vi "Automated door project by Rinat.vi"() -> ()   [LabVIEW 2020]
panel:
  out "String 2":string
  out "String":string
  in  "stop":bool
  out "Door 2":dbl(slide)
  in  "Distance from the door":dbl(knob) scale=0.2..3.0
  out "Door":dbl(slide) scale=0.0..100.0
  out "Door Motor (Closing)":bool
  out "Door Motor (Opening)":bool
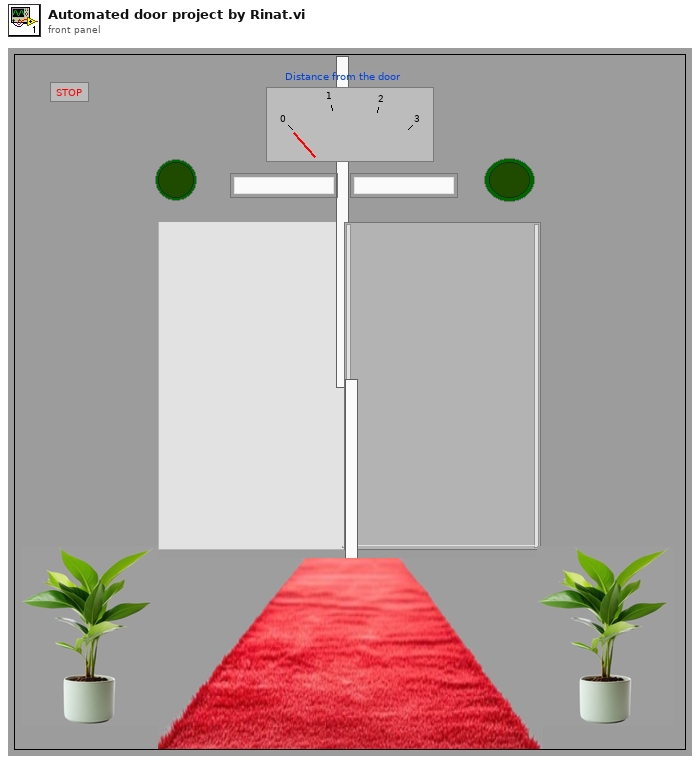
[diagram p1: front panel]
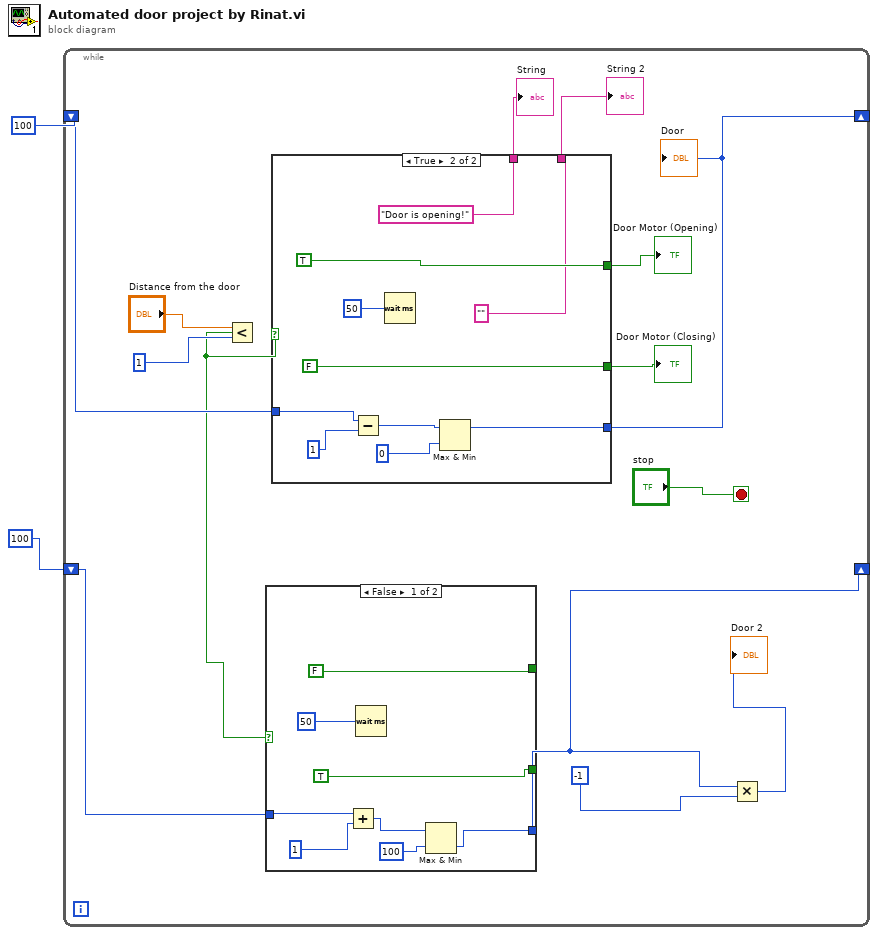
[diagram p0: block diagram]
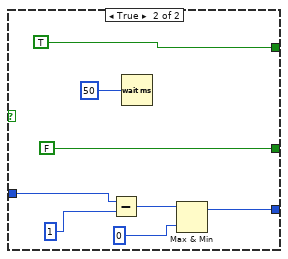
[diagram p2: hidden frame]
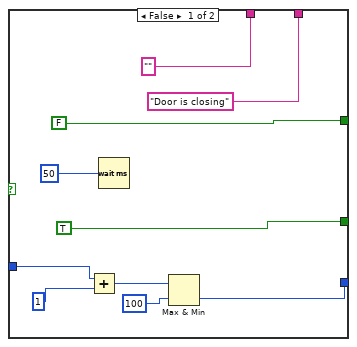
[diagram p3: hidden frame]
diagram:
  n1 = while {
    shift-right: [w14] -> _
    shift-left: 100 -> [w11]
    shift-right: [w6] -> _
    shift-left: 100 -> [w9]
    stop <- "stop" stop-if-true
    n2 = Less?(x="Distance from the door", y=1) -> (x < y?=w3:bool)
    n3 = case shown="False" w3 {
      tunnel: [FALSE TRUE] -> _
      tunnel: [TRUE FALSE] -> _
      tunnel: w9 -> [w19 w28]
      tunnel: [w20 w25] -> w6
      frame False {
        n4 = Add(x=w19, y=1) -> (x+y=w17:i32)
        n5 = Wait (ms)(milliseconds to wait=50) -> ()  [unwired: 1 out]
        n6 = Max & Min(x=w17, y=100) -> (min(x,y)=w20:i32)  [unwired: 1 out]
      }
      frame True {
        n7 = Subtract(x=w28, y=1) -> (x-y=w26:i32)
        n8 = Wait (ms)(milliseconds to wait=u32 50) -> ()  [unwired: 1 out]
        n9 = Max & Min(x=w26, y=0) -> (max(x,y)=w25:i32)  [unwired: 1 out]
      }
    }
    n10 = case shown="True" w3 {
      tunnel: [FALSE TRUE] -> w16
      tunnel: [TRUE FALSE] -> w15
      tunnel: w11 -> [w39 w49]
      tunnel: [w35 w46] -> w14
      tunnel: ["" "Door is opening!"] -> w5
      tunnel: ["Door is closing" ""] -> w4
      frame False {
        n11 = Add(x=w39, y=1) -> (x+y=w36:i32)
        n12 = Wait (ms)(milliseconds to wait=50) -> ()  [unwired: 1 out]
        n13 = Max & Min(x=w36, y=100) -> (min(x,y)=w35:i32)  [unwired: 1 out]
      }
      frame True {
        n14 = Subtract(x=w49, y=1) -> (x-y=w47:i32)
        n15 = Wait (ms)(milliseconds to wait=u32 50) -> ()  [unwired: 1 out]
        n16 = Max & Min(x=w47, y=0) -> (max(x,y)=w46:i32)  [unwired: 1 out]
      }
    }
    "Door Motor (Opening)" <- w16
    "Door Motor (Closing)" <- w15
    "Door" <- w14
    "String" <- w5
    "String 2" <- w4
    n17 = Multiply(x=w6, y=-1) -> (x*y=→"Door 2":i32)
  }
